vi "控制小灯泡.vi"() -> ()   [LabVIEW 2019]
panel:
  out "布尔 2":bool
  in  "布尔":bool
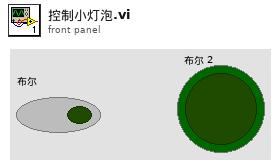
[diagram p1: front panel]
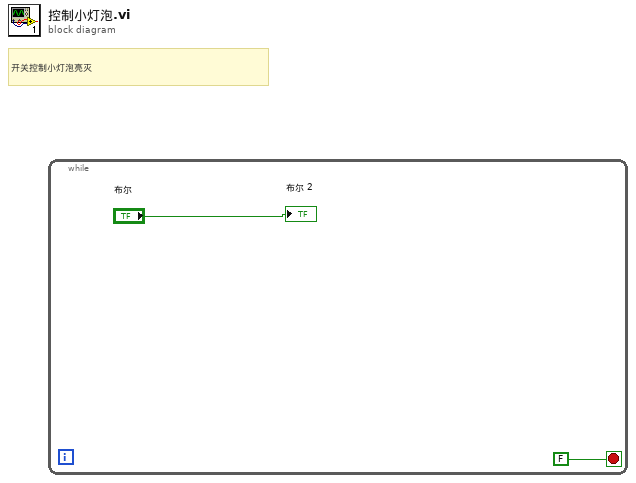
[diagram p0: block diagram]
diagram:
  # "开关控制小灯泡亮灭"
  n1 = while {
    stop <- FALSE stop-if-true
    "布尔 2" <- "布尔"
  }
